vi "Store New Theme.vi"(8 "Error In":errorcluster, 9 "Notebook Theme":T2={"Theme Name"="Light Theme", "[Named Text Styles]"=[], "Page Color"=enum."White"} {"[Named Text Styles]"."Text Formatting"."Font Size" min=6.0 step=1.0}, 11 "New Theme Name":string) -> (0 "Error Out":errorcluster, 1 "Result":T1, 3 "New Theme Name (dup)":string)   [LabVIEW 2021, in "Notebook.lvlib"]
uses:
  Notebook.lvlib
  Notebook Theme.ctl
  Rich Text Box/Named Text Style.ctl
  Rich Text Box/Text Formatting.ctl
  Rich Text Box/Text Colors.ctl
  Rich Text Box/Text Style.ctl
  Rich Text Box/Text Alignment.ctl
  Notebook Theme Edit Result.ctl
  Notebook Parameters List.ctl
  Rich Text Box/Rich Text Box.lvlib
panel:
  # "see the License on the block diagram (Ctrl+E or Window:Show Block Diagram)"
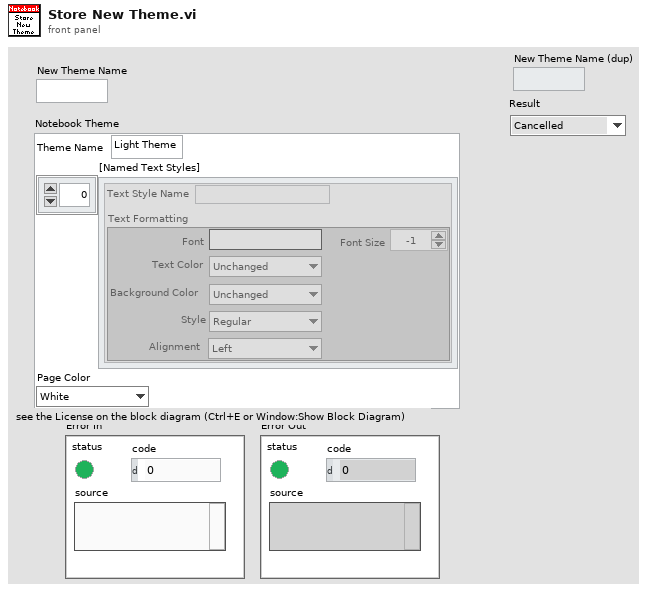
[diagram p1: front panel]
types:
  T1 = typedef "Notebook.lvlib/Notebook Theme Edit Result.ctl" = enum16{"Cancelled", "Modified Theme", "New Theme", "Remove Theme"}
  T2 = typedef "Notebook.lvlib/Notebook Theme.ctl" = cluster{"Theme Name":string, "[Named Text Styles]":T3[], "Page Color":T5}
  T3 = typedef "Notebook.lvlib/Named Text Style.ctl" = cluster{"Text Formatting":T4, "Text Style Name":string}
  T4 = typedef "Rich Text Box.lvlib/Text Formatting.ctl" = cluster{"Font":string, "Text Color":T5, "Background Color":T5, "Style":T6, "Font Size":dbl, "Alignment":T7}
  T5 = typedef "Rich Text Box.lvlib/Text Colors.ctl" = enum16{"Unchanged", "Black", "Blue", "Cyan", "Maroon", "Gray", "Violet", "Green", "Light Green", "Orange", "Yellow", "Magenta", "Red", "White"}
  T6 = typedef "Rich Text Box.lvlib/Text Style.ctl" = enum16{"Regular", "Bold", "Italic", "Underline", "Strikeout"}
  T7 = typedef "Rich Text Box.lvlib/Text Alignment.ctl" = enum16{"Left", "Right", "Center"}
  T8 = typedef "Notebook.lvlib/Notebook Parameters List.ctl" = enum16{"First Opening?", "Saved Notebook?", "Saved Notebook Path", "Beep on Error?", "Notebook Themes", "Current Theme Name"}
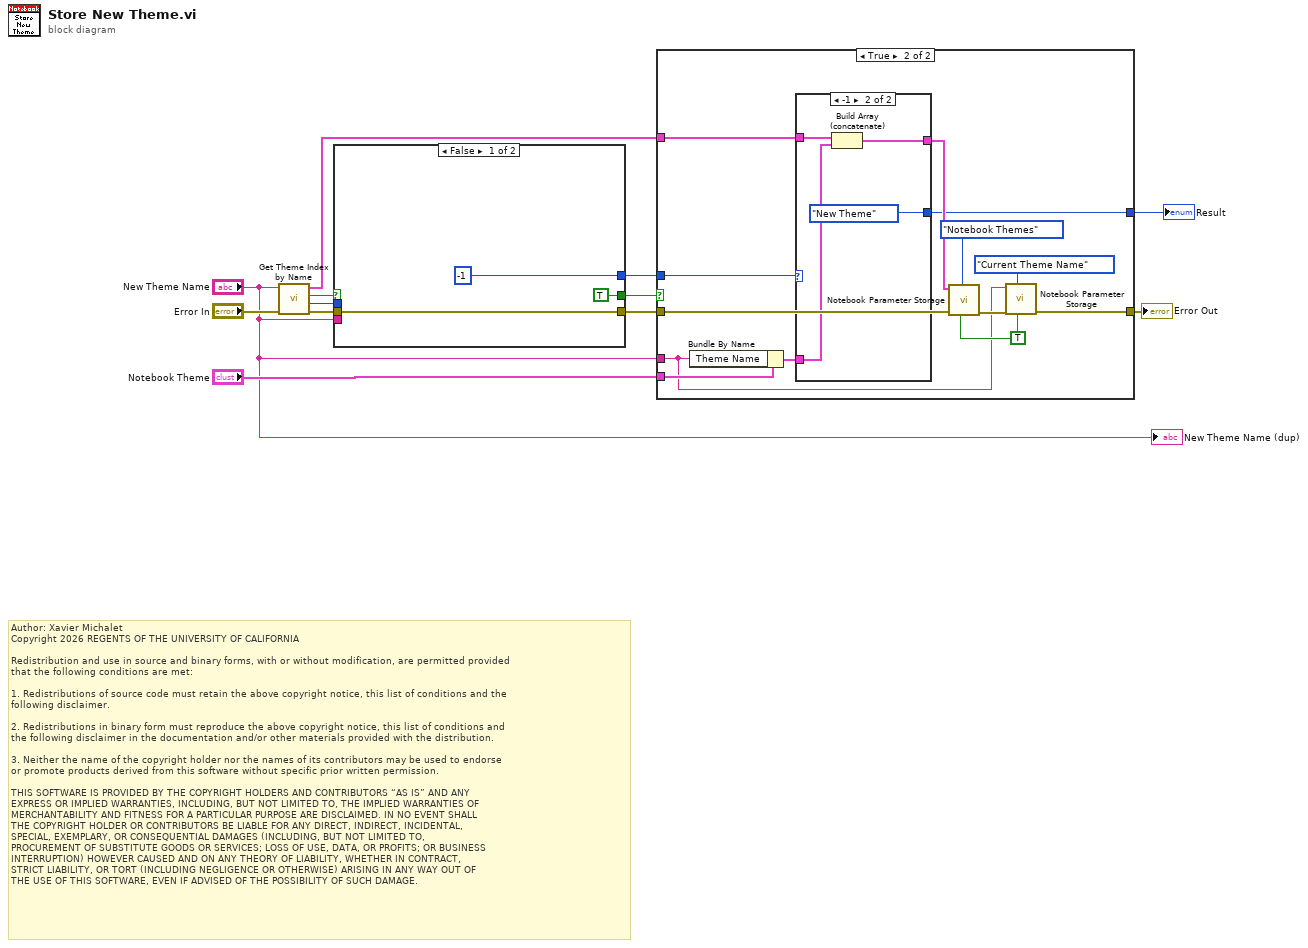
[diagram p0: block diagram]
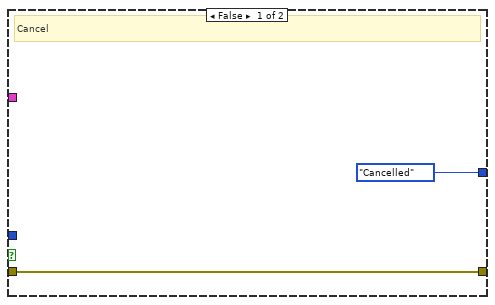
[diagram p2: hidden frame]
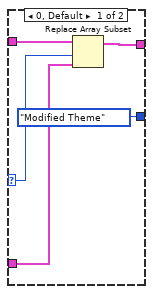
[diagram p3: hidden frame]
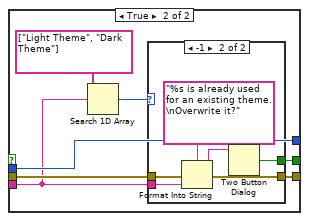
[diagram p4: hidden frame]
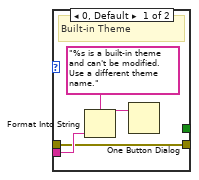
[diagram p5: hidden frame]
diagram:
  # "Author: Xavier Michalet\nCopyright 2026 REGENTS OF THE UNIVERSITY OF CALIFORNIA\n\nRedistribution and use in source and binary forms, with or without modification, are permitted provided\nthat the following conditions are met:\n\n1. Redistributions of source code must retain the above copyright notice, this list of conditions and the\nfollowing disclaimer.\n\n2. Redistributions in binary form must reproduce the above copyright notice, this list of conditions and\nthe following disclaimer in the documentation and/or other materials provided with the distribution.\n\n3. Neither the name of the copyright holder nor the names of its contributors may be used to endorse \nor promote products derived from this software without specific prior written permission.\n\nTHIS SOFTWARE IS PROVIDED BY THE COPYRIGHT HOLDERS AND CONTRIBUTORS “AS IS” AND ANY \nEXPRESS OR IMPLIED WARRANTIES, INCLUDING, BUT NOT LIMITED TO, THE IMPLIED WARRANTIES OF\nMERCHANTABILITY AND FITNESS FOR A PARTICULAR PURPOSE ARE DISCLAIMED. IN NO EVENT SHALL\nTHE COPYRIGHT HOLDER OR CONTRIBUTORS BE LIABLE FOR ANY DIRECT, INDIRECT, INCIDENTAL, \nSPECIAL, EXEMPLARY, OR CONSEQUENTIAL DAMAGES (INCLUDING, BUT NOT LIMITED TO, \nPROCUREMENT OF SUBSTITUTE GOODS OR SERVICES; LOSS OF USE, DATA, OR PROFITS; OR BUSINESS\nINTERRUPTION) HOWEVER CAUSED AND ON ANY THEORY OF LIABILITY, WHETHER IN CONTRACT, \nSTRICT LIABILITY, OR TORT (INCLUDING NEGLIGENCE OR OTHERWISE) ARISING IN ANY WAY OUT OF\nTHE USE OF THIS SOFTWARE, EVEN IF ADVISED OF THE POSSIBILITY OF SUCH DAMAGE."
  n1 = call "Get Theme Index by Name.vi"("error in (no error)"="Error In", "Theme Name"="New Theme Name") -> ("error out"=w5:errorcluster, "Theme Index"=w8:i32, "Found"=w12:bool, "Theme Array"=w10:T2[])  [unwired: 6 in]
  n2 = case shown="False" w12 {
    tunnel: "New Theme Name" -> [_ w18]
    tunnel: [TRUE ("T button?") w22] -> w11
    tunnel: w8 -> [_ w21]
    tunnel: [-1 w21] -> w7
    tunnel: w5 -> [w14 w20]
    tunnel: [w14 w19] -> w4
    frame False {
    }
    frame True {
      n3 = Search 1D Array(1D array=string[] ["Light Theme", "Dark Theme"], element=w18) -> (index of element=w16:i32)  [unwired: 1 in]
      n4 = case shown="-1" w16 {
        tunnel: w18 -> [w26 w31]
        tunnel: [_ w29] -> w22
        tunnel: w20 -> [w23 w28]
        tunnel: [w23 w27] -> w19
        frame 0, Default {
          # "Built-in Theme"
          n5 = Format Into String(format string="%s is a built-in theme and can't be modified. Use a different theme name.", w26) -> (resulting string=w24:string)  [unwired: 2 in, 1 out]
          n6 = One Button Dialog(message=w24) -> ()  [unwired: 1 in, 1 out]
        }
        frame -1 {
          n7 = Format Into String(format string="%s is already used for an existing theme.\nOverwrite it?", error in=w28, w31) -> (resulting string=w30:string, error out=w27:errorcluster)  [unwired: 1 in]
          n8 = Two Button Dialog(message=w30) -> (T button?=w29:bool)  [unwired: 2 in]
        }
      }
    }
  }
  n9 = case shown="True" w11 {
    tunnel: w10 -> [_ w44]
    tunnel: "Notebook Theme" -> [_ w46]
    tunnel: "New Theme Name" -> [_ w39]
    tunnel: w7 -> [_ w45]
    tunnel: w4 -> [w34 w38]
    tunnel: [w34 w37] -> w3
    tunnel: [Notebook_Theme_Edit_Result."Cancelled" ("Result") w36] -> w2
    frame False {
      # "Cancel"
    }
    frame True {
      w41 = TRUE ("Get(F)/Set")
      n10 = Bundle By Name(cluster=w46, "Theme Name"=w39) -> (w43:T2)
      n11 = case shown="-1" w45 {
        selector: w45 -> [w50 _]
        tunnel: w44 -> [w52 w56]
        tunnel: w43 -> [w49 w55]
        tunnel: [w51 w54] -> w42
        tunnel: [Notebook_Theme_Edit_Result."Modified Theme" ("Result") Notebook_Theme_Edit_Result."New Theme" ("Result")] -> w36
        frame 0, Default {
          n12 = Replace Array Subset(array=w52, new element=w49, index=w50) -> (w51:T2[])
        }
        frame -1 {
          n13 = Build Array (concatenate)(w56, w55) -> (w54:T2[])
        }
      }
      n14 = call "Notebook Parameter Storage.vi"("Get(F)/Set"=w41, "Notebook Parameter List"=Notebook_Parameters_List."Notebook Themes", "Error In"=w38, "Data in"=w42) -> ("Error Out"=w40:errorcluster)  [unwired: 6 in, 1 out]
      n15 = call "Notebook Parameter Storage.vi"("Get(F)/Set"=w41, "Notebook Parameter List"=Notebook_Parameters_List."Current Theme Name", "Error In"=w40, "Data in"=w39) -> ("Error Out"=w37:errorcluster)  [unwired: 6 in, 1 out]
    }
  }
  "Error Out" <- w3
  "Result" <- w2
  "New Theme Name (dup)" <- "New Theme Name"
